vi "Assert Almost Equal_Float.vi"(3 "Execution time (s)":dbl=-1.0, 4 "Use Percentage of X (F)":bool, 6 "error code (1)":i32=1, 7 "Label":string, 8 "error in":errorcluster, 9 "Tolerance":ext=0.00000100000000000000000004, 10 "Y":ext, 11 "X":ext) -> (0 "error out":errorcluster, 2 "Properties":refnum<class "Properties.Assert.lvclass">)   [LabVIEW 2021, in "Banana.Caraya.lvlib" / "Platano.CarayaTestSuite.lvclass"]
uses:
  Platano.CarayaTestSuite.lvclass
  <vilib>/addons/_JKI Toolkits/Caraya/classes/Properties.Assert/Properties.Assert.lvclass
  C:/Program Files (x86)/National Instruments/LabVIEW 2021/vi.lib/addons/_JKI Toolkits/Caraya/classes/Properties/Properties.lvclass
  Bananas/Banana/Banana.lvclass/Banana.ctl
  Bananas/AssertAlmostEqual/AssertAlmostEqualValue.lvclass/AssertAlmostEqualValue.ctl
  Bananas/AssertAlmostEqual/Write X.vi
  Bananas/AssertAlmostEqual/Write Y.vi
  Bananas/AssertAlmostEqual/Write Tolerance.vi
  Bananas/AssertAlmostEqual/Write Pct_of_X.vi
  <vilib>/LabVIEW Open Source Project/Data Manipulation/Variant/Variant_SetName.vi
  <vilib>/LabVIEW Open Source Project/Data Manipulation/Variant/Variant_BuildClusterFromElementArray.vi
  Bananas/Banana/Read Ephemerals.vi
  <vilib>/LabVIEW Open Source Project/Data Manipulation/Variant/Variant_EmptyCluster.vi
  Bananas/AssertAlmostEqual/AssertAlmostEqualValue.lvclass
  C:/Repositories/LVOS/Bananas/lv-src/Bananas/BananaPeel/BananaPeel.lvclass
  <vilib>/addons/_JKI Toolkits/Caraya/classes/Assert/Assert True.vi
  <vilib>/LabVIEW Open Source Project/Data Manipulation/Variant/Variant_ListElements.vi
  <vilib>/LabVIEW Open Source Project/Data Manipulation/TypeDescriptor/TypeDescriptor_SetName.vi
  <vilib>/Utility/GetType.llb/TD_Create Cluster.vi
  Bananas/AssertTrue/AssertTrue.lvclass
  Bananas/AssertFalse/AssertFalse.lvclass
  Bananas/AssertEqualValue/AssertEqualValue.lvclass
  Bananas/AssertEqualType/AssertEqualType.lvclass
  Bananas/AssertCompareValue/AssertCompareValue.lvclass
  Bananas/AssetError/AssertError.lvclass
  Bananas/BananaPeel/BananaPeel.lvclass
  <vilib>/addons/_JKI Toolkits/Caraya/classes/Assert/Assert.lvclass
  Bananas/Platano/Platano.lvclass
  Bananas/Banana/Banana.lvclass
  Properties.Banana/Properties.Banana.lvclass
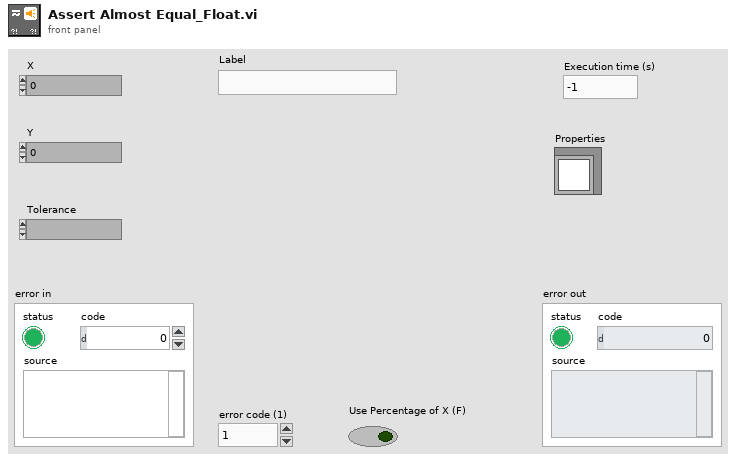
[diagram p1: front panel]
types:
  T1 = typedef "Bananas.lvlib/Assertion Strategies -- cluster.ctl" = cluster{"AssertTrue":refnum<class "AssertTrue.lvclass">, "AssertFalse":refnum<class "AssertFalse.lvclass">, "AssertEqualValue":refnum<class "AssertEqualValue.lvclass">, "AssertEqualType":refnum<class "AssertEqualType.lvclass">, "AssertCompareValue":refnum<class "AssertCompareValue.lvclass">, "AssertError":refnum<class "AssertError.lvclass">, "AssertAlmostEqual":refnum<class "AssertAlmostEqualValue.lvclass">}
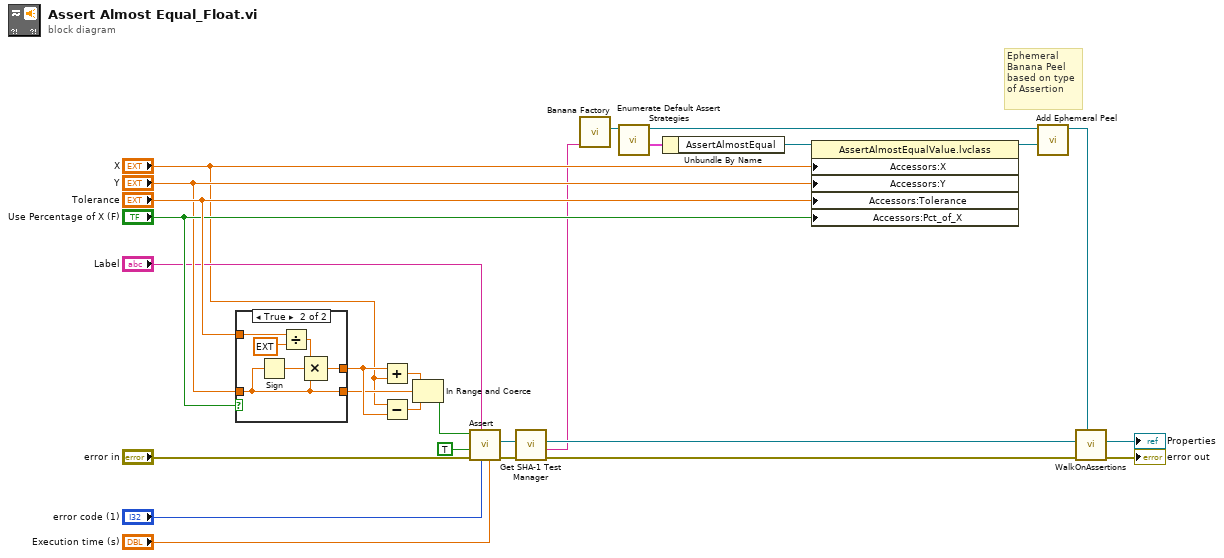
[diagram p0: block diagram]
diagram:
  # "Ephemeral\nBanana Peel\nbased on type\nof Assertion"
  n1 = case shown="True" "Use Percentage of X (F)" {
    tunnel: "Tolerance" -> [w29 w35]
    tunnel: [w29 w32] -> w18
    tunnel: "Y" -> [w28 w31]
    tunnel: [w28 w31] -> w17
    frame False {
    }
    frame True {
      n2 = Sign(1:w31) -> (0:w33:ext)
      n3 = Divide(x=w35, y=ext 100.0) -> (x/y=w30:ext)
      n4 = Compound Arithmetic op=MULTIPLY(w30, w33, w31) -> (w32:ext)
    }
  }
  n5 = Add(x=w18, y="X") -> (x+y=w20:ext)
  n6 = Subtract(x="X", y=w18) -> (x-y=w19:ext)
  n7 = In Range and Coerce(upper limit=w20, x=w17, lower limit=w19) -> (In Range?=w13:bool)  [unwired: 1 out]
  n8 = call-poly <vilib>:"Assert.vi"("Execution time (s)"="Execution time (s)", "error code (1)"="error code (1)", "Label"="Label", "error in (no error)"="error in", "Register with caller test (F)"=TRUE, "True?"=w13) -> ("error out"=w6:errorcluster, "Properties"=w3:refnum<class "Properties.Assert.lvclass">)  [unwired: 4 in]
  n9 = call "Get SHA-1 Test Manager.vi"("error in (no error)"=w6, "Properties"=w3) -> ("error out"=w5:errorcluster, "SHA-1 hash"=w2:string, "Properties"=w4:refnum<class "Properties.Assert.lvclass">)  [unwired: 7 in]
  n10 = call "Banana Factory.vi"("Varietal"=w2) -> ("Banana"=w1:refnum<class "Banana.lvclass">)  [unwired: 9 in, 1 out]
  n11 = call "Enumerate Default Assert Strategies.vi"("Banana"=w1) -> ("Strategies"=w23:T1, "Banana"=w24:refnum<class "Banana.lvclass">)  [unwired: 9 in]
  n12 = Unbundle By Name(w23) -> ("AssertAlmostEqual"=w22:refnum<class "AssertAlmostEqualValue.lvclass">)
  n13 = property class="AssertAlmostEqualValue.lvclass"(reference=w22, "Accessors:X"="X", "Accessors:Y"="Y", "Accessors:Tolerance"="Tolerance", "Accessors:Pct_of_X"="Use Percentage of X (F)") -> (reference out=w21:refnum<class "AssertAlmostEqualValue.lvclass">)  [unwired: 1 in, 1 out]
  n14 = call "Add Ephemeral Peel.vi"("BananaPeel"=w21, "Banana"=w24) -> ("Banana"=w25:refnum<class "Banana.lvclass">)  [unwired: 9 in]
  n15 = call "WalkOnAssertions.vi"("Banana"=w25, "error in (no error)"=w5, "Properties"=w4) -> ("error out"=→"error out":errorcluster, "Properties out"=→"Properties":refnum<class "Properties.Assert.lvclass">)  [unwired: 7 in]
